vi "ODE-CircuitRHS.vi"(2 "data":variant, 3 "t":dbl, 4 "x1, x2,...":dbl[](array[numeric])) -> (0 "error out":errorcluster, 1 "f'(x)":dbl[](array[numeric]))   [LabVIEW 2023]
doc: "This VI contains the formula of the Circuit ODE system model to be called by reference by the polymorphic ODE solver in VI mode. The Circuit system can be described by the following equations:\n\ndi2/dt = (-(R1+R2)i2 - R1i3 + Vin)/L1\ndi3/dt = (-R1i2 - R1i3 + Vin)/L2"
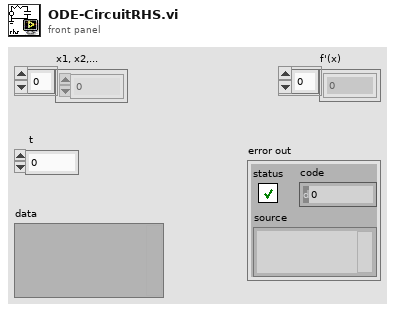
[diagram p1: front panel]
types:
  T1 = cluster{"R1":dbl, "R2":dbl, "L1":dbl, "L2":dbl, "Vin":dbl}
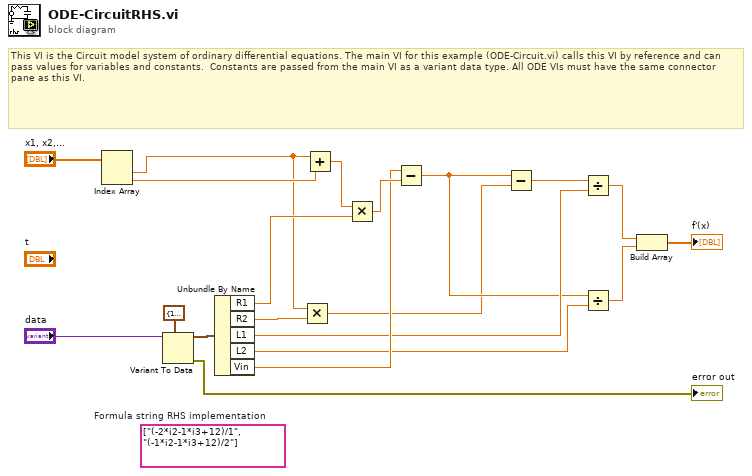
[diagram p0: block diagram]
diagram:
  (unwired) string[] ["(-2*i2-1*i3+12)/1", "(-1*i2-1*i3+12)/2"]  # Formula string RHS implementation
  # "This VI is the Circuit model system of ordinary differential equations. The main VI for this example (ODE-Circuit.vi) calls this VI by reference and can pass values for variables and constants.  Constants are passed from the main VI as a variant data type. All ODE VIs must have the same connector pane as this VI."
  n1 = Index Array(array="x1, x2,...") -> (element #1=w2:dbl, element #2=w15:dbl)  [unwired: 2 in]
  n2 = Variant To Data(type=T1 {"R1"=1.0, "R2"=1.2, "L1"=1.0, "L2"=2.0, "Vin"=12.0} ("Constants"), Variant="data") -> (data=w17:T1, error out=→"error out":errorcluster)  [unwired: 1 in]
  n3 = Unbundle By Name(w17) -> ("R1"=w13:dbl, "R2"=w7:dbl, "L1"=w8:dbl, "L2"=w10:dbl, "Vin"=w11:dbl)
  n4 = Multiply(x=w2, y=w7) -> (x*y=w5:dbl)
  n5 = Add(x=w2, y=w15) -> (x+y=w14:dbl)
  n6 = Multiply(x=w14, y=w13) -> (x*y=w12:dbl)
  n7 = Subtract(x=w11, y=w12) -> (x-y=w6:dbl)
  n8 = Subtract(x=w6, y=w5) -> (x-y=w4:dbl)
  n9 = Divide(x=w4, y=w8) -> (x/y=w3:dbl)
  n10 = Divide(x=w6, y=w10) -> (x/y=w9:dbl)
  n11 = Build Array(w3, w9) -> (→"f'(x)":dbl[])
